vi "Test Method Result Has Test Name.vi"(8 "error in (no error)":errorcluster, 11 "Pass Assertion Test In":refnum<class "Method Result Test.lvclass">) -> (0 "error out":errorcluster, 3 "Pass Assertion Test Out":refnum<class "Method Result Test.lvclass">)   [LabVIEW 2020, in "LUnit Tests.lvlib" / "Method Result Test.lvclass"]
uses:
  Method Result Test.lvclass
  Method Result Test.lvclass/Method Result Test.ctl
  2ab93ff3-45be-4610-b1ef-bc0fe70d6813.vi
  56e160e8-8c04-4a76-96a9-5548a9139eef.vi
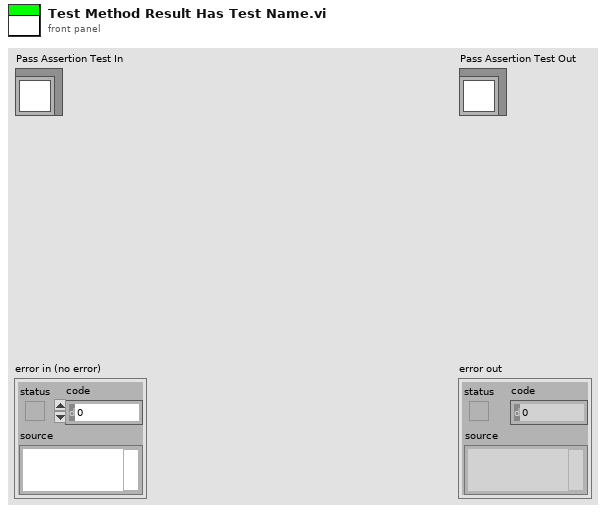
[diagram p1: front panel]
types:
  T1 = typedef "Method Result.lvlib/Method Result.ctl" = cluster{"Test Case":string, "Test Method Name":string, "Status":T2, "Assertion Results":T3[], "Execution time":dbl, "Result String":string}
  T2 = typedef "Assertion Result.lvlib/Status.ctl" = enum16{"Pass", "Fail", "Error", "Skipped", "Setup Error", "Broken", "Teardown Error"}
  T3 = typedef "Assertion Result.lvlib/Assertion Result.ctl" = cluster{"Status":T2, "Message":string, "Description":string, "Assertion Type":T4}
  T4 = typedef "Assertion Result.lvlib/Assertion Type.ctl" = enum16{"None", "Pass", "Fail", "Skip", "Pass if Equal", "Fail if Equal", "Pass if Error", "Fail if Error", "Pass if", "Fail if"}
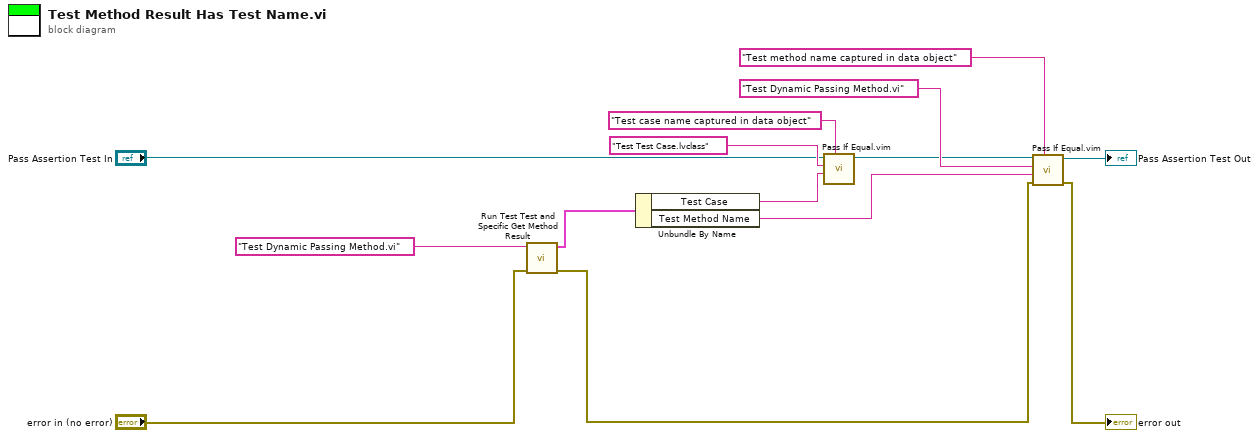
[diagram p0: block diagram]
diagram:
  n1 = call "Run Test Test and Specific Get Method Result.vi"("error in (no error)"="error in (no error)", "Method of Interest"="Test Dynamic Passing Method.vi") -> ("error out"=w5:errorcluster, "Method Result out"=w3:T1)  [unwired: 8 in]
  n2 = Unbundle By Name(w3) -> ("Test Case"=w2:string, "Test Method Name"=w1:string)
  n3 = call "Pass If Equal.vim"("Description"="Test case name captured in data object", "Actual"=w2, "Expected"="Test Test Case.lvclass", "LUnit Test Case In"="Pass Assertion Test In") -> ("LUnit Test Case Out"=w8:refnum<class "Method Result Test.lvclass">)  [unwired: 6 in, 1 out]
  n4 = call "Pass If Equal.vim"("Description"="Test method name captured in data object", "error in (no error)"=w5, "Actual"=w1, "Expected"="Test Dynamic Passing Method.vi", "LUnit Test Case In"=w8) -> ("error out"=→"error out":errorcluster, "LUnit Test Case Out"=→"Pass Assertion Test Out":refnum<class "Method Result Test.lvclass">)  [unwired: 5 in]
